vi "VCA_Out.vi"(6 "Scale":i8, 9 "Sample In":fxp<+/-,8,8>) -> (1 "Sample Out":i16)   [LabVIEW 2015]
doc: "Amplifies or attenuates the input sample by performing a simple bitwise operation."
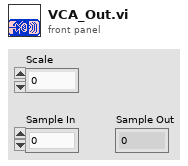
[diagram p1: front panel]
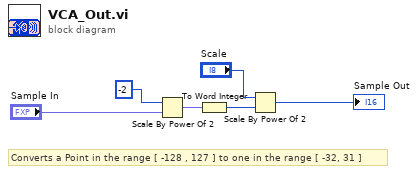
[diagram p0: block diagram]
diagram:
  # "Converts a Point in the range [ -128 , 127 ] to one in the range [ -32, 31 ]"
  n1 = Scale By Power Of 2(n=i8 -2, x="Sample In") -> (x*2^n=w1:fxp<+/-,8,8>)
  n2 = To Word Integer(number=w1) -> (16bit integer=w4:i16)
  n3 = Scale By Power Of 2(n="Scale", x=w4) -> (x*2^n=→"Sample Out":i16)
